vi "simple.vi"() -> (3 "Numeric":i32)   [LabVIEW 2012]
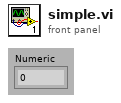
[diagram p1: front panel]
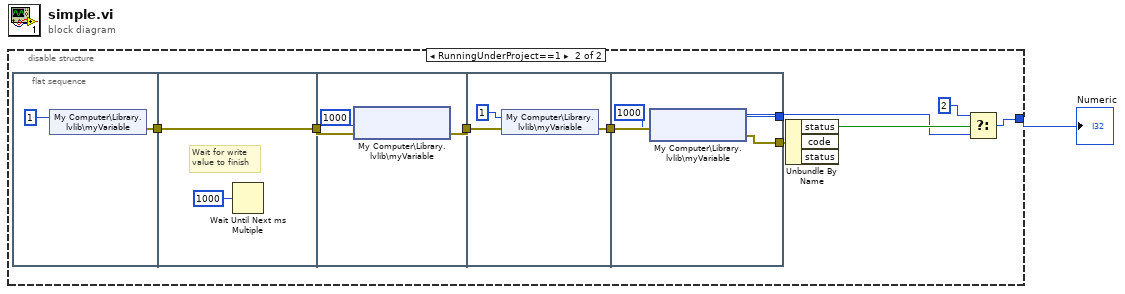
[diagram p0: block diagram]
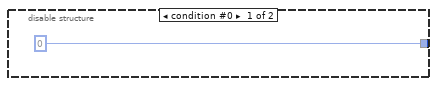
[diagram p2: hidden frame]
diagram:
  n1 = disable-structure shown="RunningUnderProject==1" {
    disable-tunnel: [0 w6] -> w1
    frame condition #0 {
    }
    frame condition #1 (active) {
      n2 = flat-sequence {
        tunnel: [w12] -> w4
        tunnel: w4 -> [w15]
        tunnel: [w15] -> w3
        tunnel: w3 -> [w18]
        tunnel: [w17] -> w5
        tunnel: [w21] -> w11
        tunnel: w5 -> [w19]
        tunnel: w11 -> [w25]
        tunnel: [w24] -> w7
        tunnel: [w23] -> w10
        frame #0 {
          n3 = shared-variable "My Computer\\Library.lvlib\\myVariable"(1 ("Numeric")) -> (error out=w12:errorcluster)  [unwired: 1 in]
        }
        frame #1 {
          # "Wait for write\nvalue to finish"
          n4 = Wait Until Next ms Multiple(millisecond multiple=u32 1000) -> ()  [unwired: 1 out]
        }
        frame #2 {
          n5 = shared-variable "My Computer\\Library.lvlib\\myVariable"(error in=w18, 1000 ("ms timeout (0)")) -> (error out=w17:errorcluster)  [unwired: 2 out]
        }
        frame #3 {
          n6 = shared-variable "My Computer\\Library.lvlib\\myVariable"(1 ("Numeric"), error in=w19) -> (error out=w21:errorcluster)
        }
        frame #4 {
          n7 = shared-variable "My Computer\\Library.lvlib\\myVariable"(error in=w25, 1000 ("ms timeout (0)")) -> (w24:i32, error out=w23:errorcluster)  [unwired: 1 out]
        }
      }
      n8 = Unbundle By Name(w10) -> ("status"=w9:bool)  [unwired: 2 out]
      n9 = Select(t=2 ("Numeric"), s=w9, f=w7) -> (s? t:f=w6:i32)
    }
  }
  "Numeric" <- w1
